vi "CoreSNF.vi"() -> (19 "Error Out":errorcluster)   [LabVIEW 2017]
uses:
  <vilib>/Platform/TimedLoop/XDataNode/XDataNode.xnode
  <vilib>/Platform/TimedLoop/XDataNode/nitl_modes.ctl
  <vilib>/Platform/TimedLoop/XDataNode/XDNodeRunTimeDep.lvlib
  <vilib>/Platform/TimedLoop/XDataNode/wakeup.ctl
  <vilib>/Platform/TimedLoop/XDataNode/timing_clust.ctl
panel:
  out "Output Resistance 3":dbl
  out "Output Resistance":dbl
  # "Core Module DIagnostics"
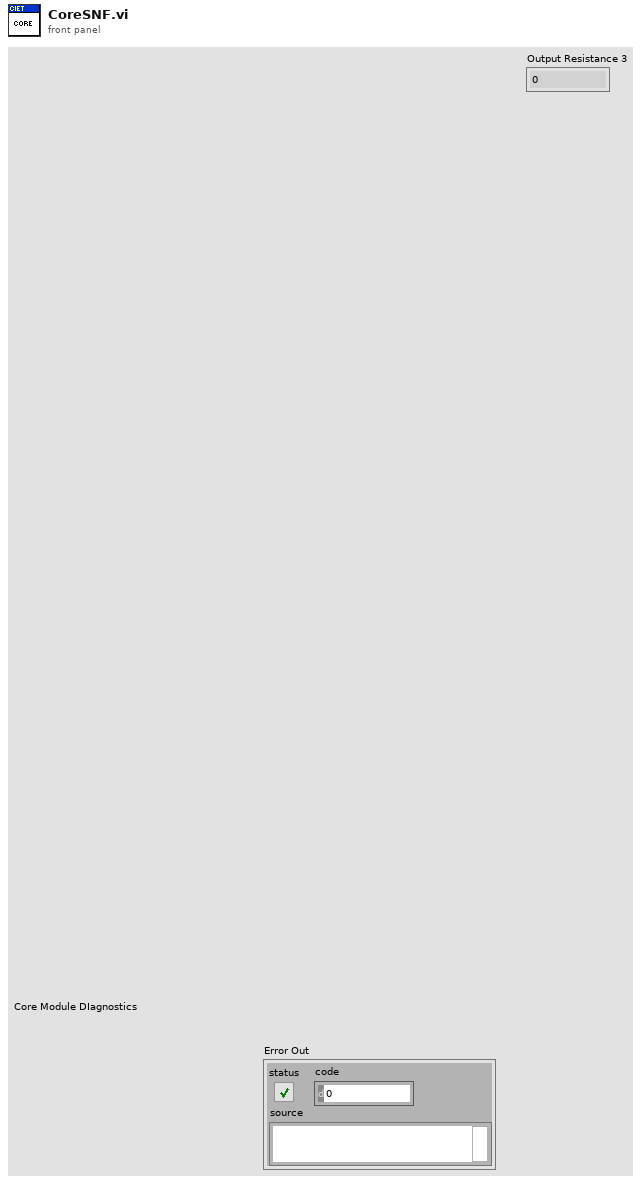
[diagram p1: front panel]
types:
  T1 = typedef "XDNodeRunTimeDep.lvlib/timing_clust.ctl" = cluster{"Expected End [f-1]":u64, "Actual End [f-1]":u64, "Finished Late? [f-1]":bool, "Expected End [i-1]":u64, "Actual End [i-1]":u64, "Finished Late? [i-1]":bool, "Expected Start [i]":u64, "Actual Start [i]":u64, "Expected Start [f]":u64, "Actual Start [f]":u64, "Source Name":string, "Structure Name":string, "Period":i64, "Deadline":i64, "Offset":i64, "Start":i64, "Priority":i32, "Timeout":i32, "Mode":T2, "Wakeup Reason":T3, "Error":errorcluster, "Source Type":string, "Secondary Source Type":string, "Global End Time":u64, "Global Start Time":u64, "Frame Duration":u64, "Iteration Duration":u64, "Assigned CPU":i32, "I/O Scan Engine Mode":u32}
  T2 = typedef "XDNodeRunTimeDep.lvlib/nitl_modes.ctl" = enum32{"No Change", "Process missed periods, maintain original phase", "Discard missed periods, maintain original phase", "Process missed periods, ignore original phase", "Discard missed periods, ignore original phase"}
  T3 = typedef "XDNodeRunTimeDep.lvlib/wakeup.ctl" = enum32{"Normal", "Aborted", "Asynchronous wakeup", "Timing source error", "Timed loop error", "Timeout"}
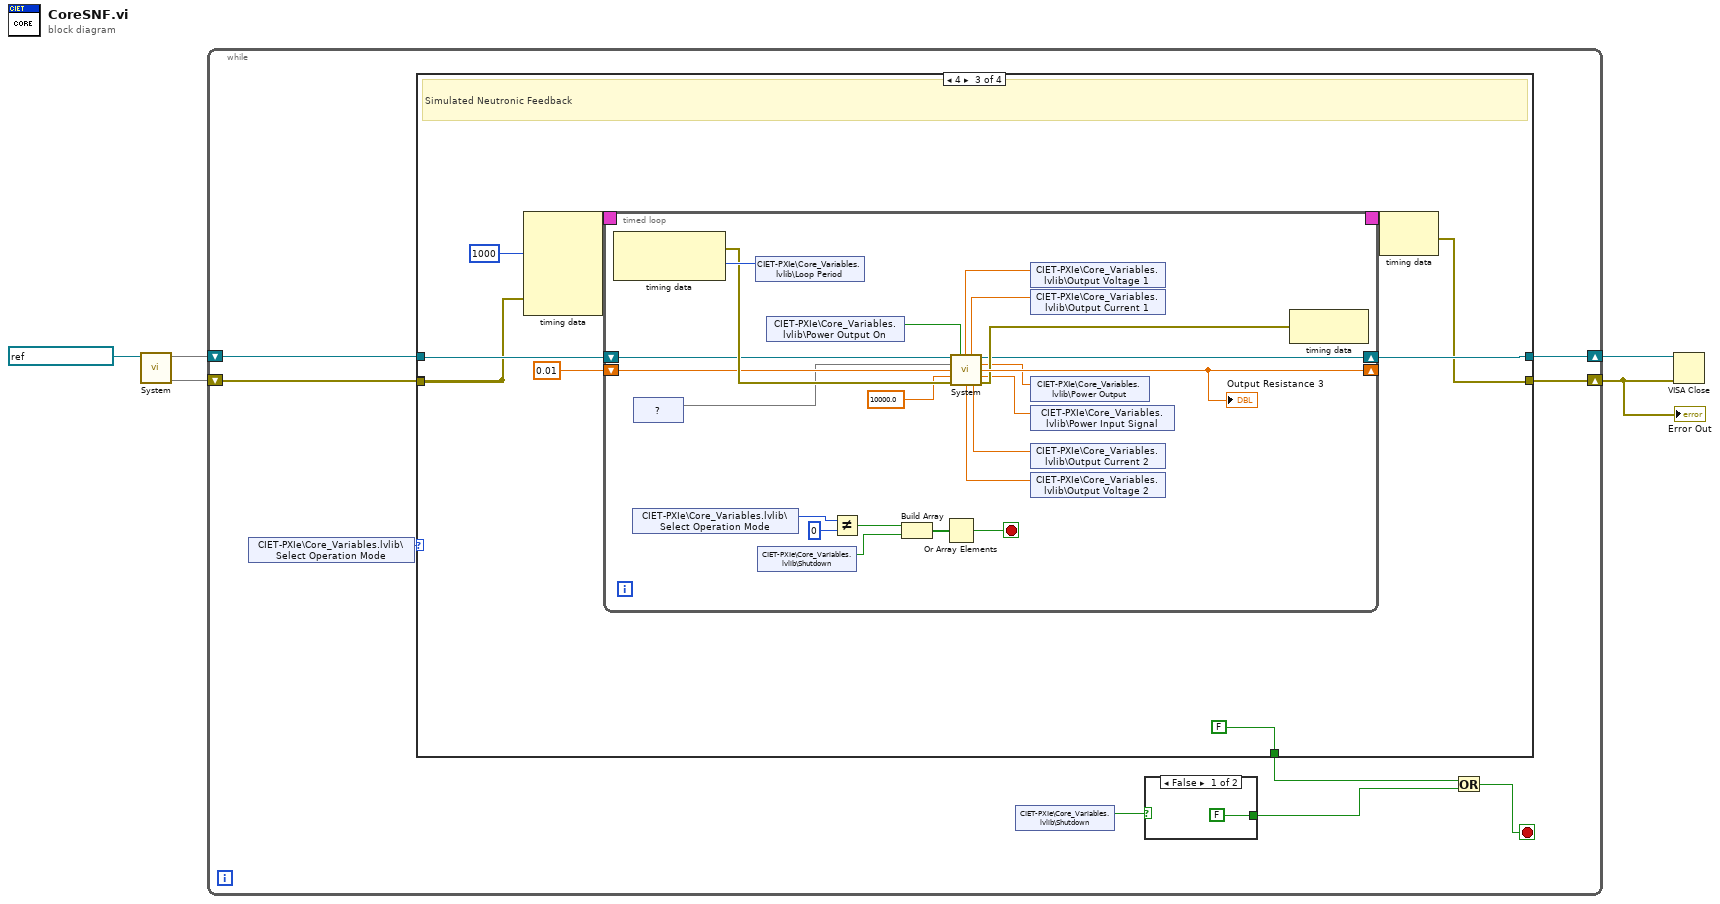
[diagram p0: block diagram]
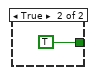
[diagram p2: hidden frame]
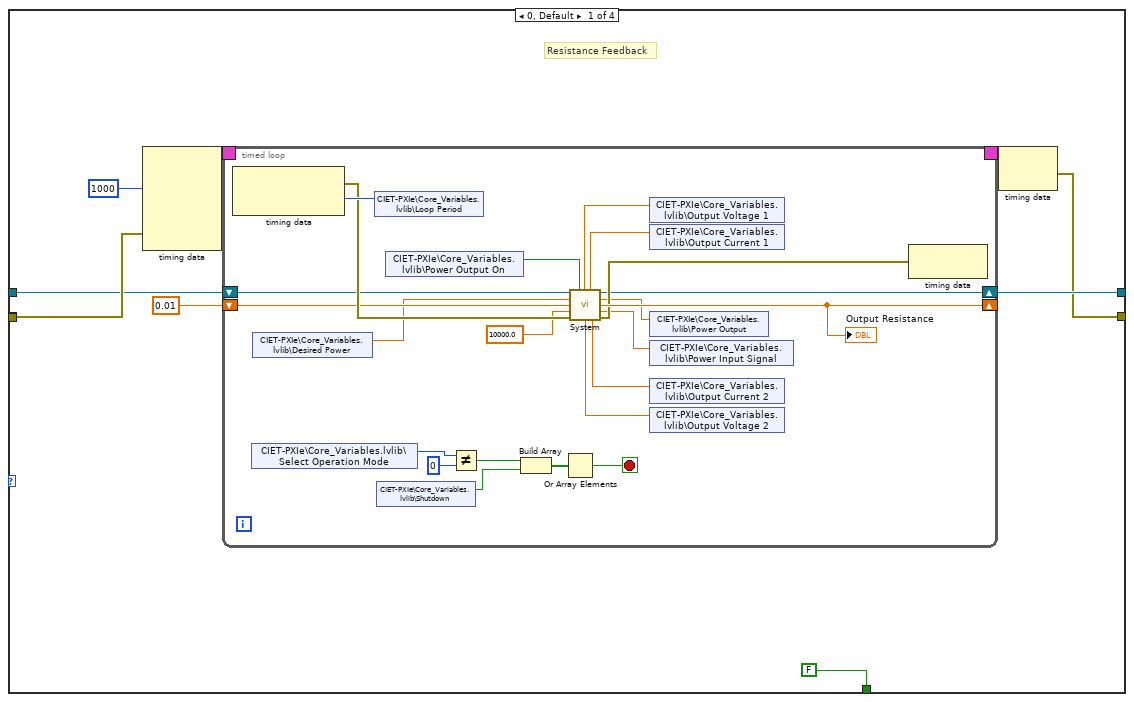
[diagram p3: hidden frame]
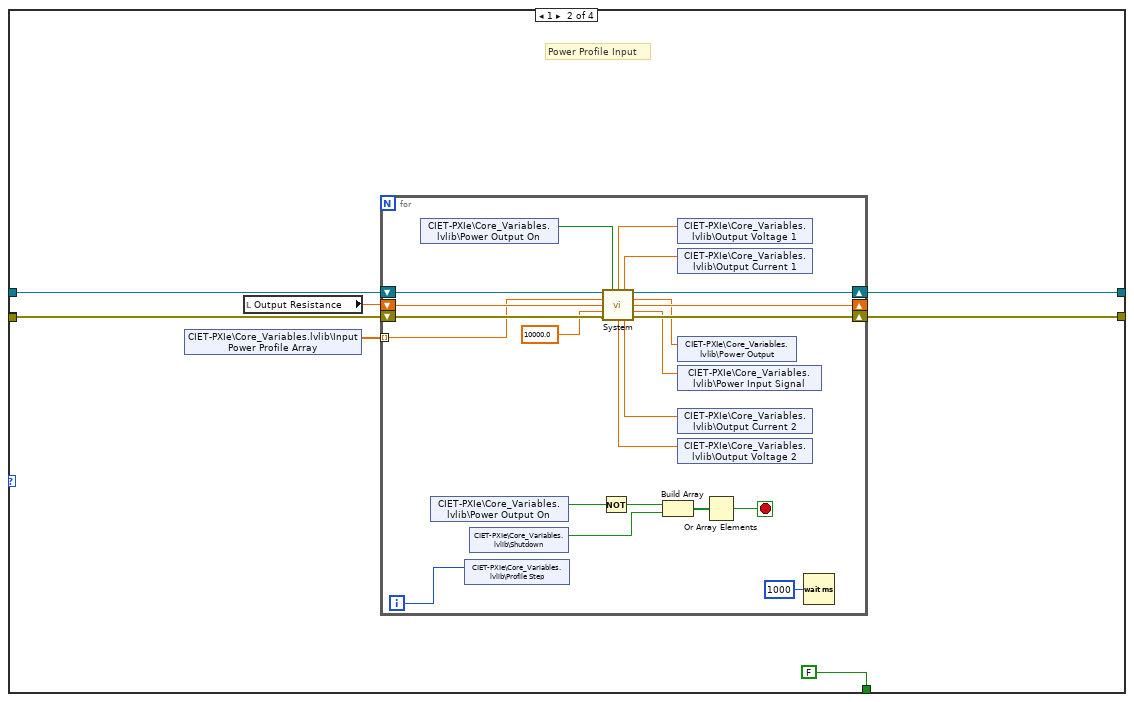
[diagram p4: hidden frame]
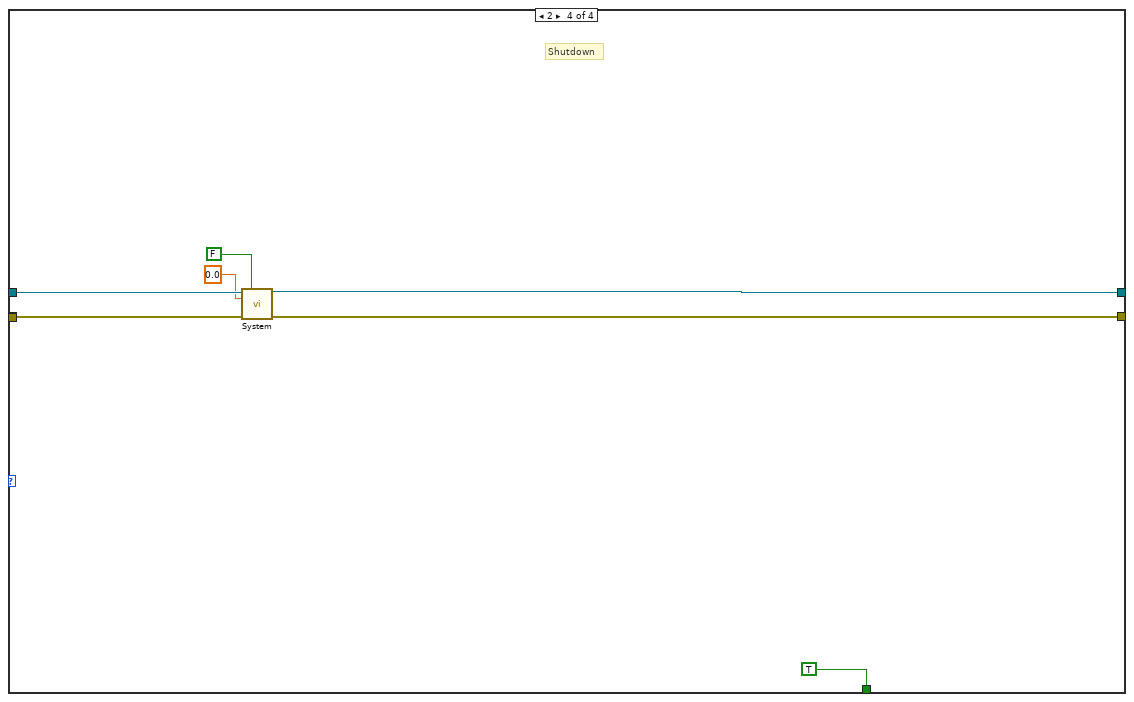
[diagram p5: hidden frame]
diagram:
  n1 = call "System.vi"(11:refnum<visa-resource-name> "PowerSupplies" ("VISA name")) -> (0:w1, 3:w2)  [unwired: 9 in]
  n2 = while {
    shift-right: [w11] -> w4
    shift-left: w1 -> [w14]
    shift-right: [w12] -> w5
    shift-left: w2 -> [w13]
    stop <- w6 stop-if-true
    n3 = shared-variable "CIET-PXIe\\Core_Variables.lvlib\\Select Operation Mode"() -> (w10:i32)  [unwired: 1 in, 1 out]
    n4 = case shown="4" w10 {
      tunnel: w14 -> [w23 w63 w92 w137]
      tunnel: w13 -> [w22 w66 w93 w136]
      tunnel: [w20 w65 w91 w135] -> w12
      tunnel: [w19 w62 w90 w134] -> w11
      tunnel: [FALSE ("Shutdown") FALSE ("Shutdown") FALSE ("Shutdown") TRUE ("Shutdown")] -> w8
      tunnel: [_ _ w92 _] -> _
      frame 0, Default {
        # "Resistance Feedback"
        n5 = node-c288(i64 1000 ("Period"), w23) -> (w25:T1)  [unwired: 3 in]
        n6 = timed-loop {
          timing: w25 -> [_]
          timing-out: [_] -> w24
          shift-right: [w32] -> w20
          shift-left: w22 -> [w39]
          shift-right: [w36] -> _
          shift-left: 0.01 -> [w38]
          stop <- w44 stop-if-true
          n7 = node-c288() -> (w40:errorcluster, w43:i64)  [unwired: 1 in]
          n8 = shared-variable "CIET-PXIe\\Core_Variables.lvlib\\Select Operation Mode"() -> (w42:i32)  [unwired: 1 in, 1 out]
          n9 = shared-variable "CIET-PXIe\\Core_Variables.lvlib\\Desired Power"() -> (w26:dbl)  [unwired: 1 in, 1 out]
          n10 = shared-variable "CIET-PXIe\\Core_Variables.lvlib\\Loop Period"(w43) -> ()  [unwired: 1 in, 1 out]
          n11 = shared-variable "CIET-PXIe\\Core_Variables.lvlib\\Shutdown"() -> (w41:bool)  [unwired: 1 in, 1 out]
          n12 = shared-variable "CIET-PXIe\\Core_Variables.lvlib\\Power Output On"() -> (w31:bool)  [unwired: 1 in, 1 out]
          n13 = Not Equal?(x=w42, y=u16 0) -> (x != y?=w46:bool)
          n14 = Build Array(w46, w41) -> (w45:bool[])
          n15 = Or Array Elements(Boolean array=w45) -> (logical OR=w44:bool)
          n16 = call "System.vi"("Input VISA"=w39, "Power Output ON"=w31, "Desired Power"=w26, "Input Resistance"=w38, "Maximum Power Limit"=10000.0, "Input Error"=w40) -> ("Output Voltage 1"=w30:dbl, "Output Current 1"=w29:dbl, "Output VISA"=w32:refnum<visa-resource-name>, "Output Power"=w33:dbl, "Output Resistance"=w36:dbl, "Input Power"=w34:dbl, "Output Voltage 2"=w27:dbl, "Output Current 2"=w28:dbl, "Output Error"=w35:errorcluster)  [unwired: 1 in]
          "Output Resistance" <- w36
          n17 = shared-variable "CIET-PXIe\\Core_Variables.lvlib\\Output Voltage 1"(w30) -> ()  [unwired: 1 in, 1 out]
          n18 = shared-variable "CIET-PXIe\\Core_Variables.lvlib\\Output Current 1"(w29) -> ()  [unwired: 1 in, 1 out]
          n19 = shared-variable "CIET-PXIe\\Core_Variables.lvlib\\Power Output"(w33) -> ()  [unwired: 1 in, 1 out]
          n20 = shared-variable "CIET-PXIe\\Core_Variables.lvlib\\Power Input Signal"(w34) -> ()  [unwired: 1 in, 1 out]
          n21 = shared-variable "CIET-PXIe\\Core_Variables.lvlib\\Output Current 2"(w28) -> ()  [unwired: 1 in, 1 out]
          n22 = shared-variable "CIET-PXIe\\Core_Variables.lvlib\\Output Voltage 2"(w27) -> ()  [unwired: 1 in, 1 out]
          n23 = node-c288(w35) -> ()  [unwired: 1 out]
        }
        n24 = node-c288(w24) -> (w19:errorcluster)
      }
      frame 1 {
        # "Power Profile Input"
        n25 = shared-variable "CIET-PXIe\\Core_Variables.lvlib\\Input Power Profile Array"() -> (w60:dbl[])  [unwired: 1 in, 1 out]
        n26 = local read "Output Resistance"() -> (w64:dbl)
        n27 = for {
          shift-right: [w80] -> w65
          shift-left: w66 -> [w81]
          shift-right: [w79] -> w62
          shift-left: w63 -> [w78]
          tunnel: w60 -> [w70] mode=indexing
          shift-right: [w72] -> _
          shift-left: w64 -> [w71]
          i -> [w82]
          stop <- w86 stop-if-true
          n28 = shared-variable "CIET-PXIe\\Core_Variables.lvlib\\Power Output On"() -> (w77:bool)  [unwired: 1 in, 1 out]
          n29 = shared-variable "CIET-PXIe\\Core_Variables.lvlib\\Power Output On"() -> (w84:bool)  [unwired: 1 in, 1 out]
          n30 = shared-variable "CIET-PXIe\\Core_Variables.lvlib\\Profile Step"(w82) -> ()  [unwired: 1 in, 1 out]
          n31 = shared-variable "CIET-PXIe\\Core_Variables.lvlib\\Shutdown"() -> (w83:bool)  [unwired: 1 in, 1 out]
          n32 = Not(x=w84) -> (.not. x?=w85:bool)
          n33 = call "System.vi"("Input VISA"=w81, "Power Output ON"=w77, "Desired Power"=w70, "Input Resistance"=w71, "Maximum Power Limit"=10000.0, "Input Error"=w78) -> ("Output Voltage 1"=w76:dbl, "Output Current 1"=w75:dbl, "Output VISA"=w80:refnum<visa-resource-name>, "Output Power"=w68:dbl, "Output Resistance"=w72:dbl, "Input Power"=w67:dbl, "Output Voltage 2"=w74:dbl, "Output Current 2"=w73:dbl, "Output Error"=w79:errorcluster)  [unwired: 1 in]
          n34 = Build Array(w85, w83) -> (w88:bool[])
          n35 = shared-variable "CIET-PXIe\\Core_Variables.lvlib\\Output Voltage 1"(w76) -> ()  [unwired: 1 in, 1 out]
          n36 = shared-variable "CIET-PXIe\\Core_Variables.lvlib\\Output Current 1"(w75) -> ()  [unwired: 1 in, 1 out]
          n37 = shared-variable "CIET-PXIe\\Core_Variables.lvlib\\Power Output"(w68) -> ()  [unwired: 1 in, 1 out]
          n38 = shared-variable "CIET-PXIe\\Core_Variables.lvlib\\Power Input Signal"(w67) -> ()  [unwired: 1 in, 1 out]
          n39 = shared-variable "CIET-PXIe\\Core_Variables.lvlib\\Output Current 2"(w73) -> ()  [unwired: 1 in, 1 out]
          n40 = shared-variable "CIET-PXIe\\Core_Variables.lvlib\\Output Voltage 2"(w74) -> ()  [unwired: 1 in, 1 out]
          n41 = Or Array Elements(Boolean array=w88) -> (logical OR=w86:bool)
          n42 = Wait (ms)(milliseconds to wait=u32 1000) -> ()  [unwired: 1 out]
        }
      }
      frame 4 {
        # "Simulated Neutronic Feedback"
        n43 = node-c288(i64 1000 ("Period"), w92) -> (w97:T1)  [unwired: 3 in]
        n44 = timed-loop {
          timing: w97 -> [_]
          timing-out: [_] -> w96
          shift-right: [w104] -> w91
          shift-left: w93 -> [w111]
          shift-right: [w108] -> _
          shift-left: 0.01 -> [w110]
          stop <- w116 stop-if-true
          n45 = node-c288() -> (w112:errorcluster, w115:i64)  [unwired: 1 in]
          n46 = shared-variable "CIET-PXIe\\Core_Variables.lvlib\\Select Operation Mode"() -> (w114:i32)  [unwired: 1 in, 1 out]
          n47 = shared-variable "?"() -> (w98)  [unwired: 1 in, 1 out]
          n48 = shared-variable "CIET-PXIe\\Core_Variables.lvlib\\Loop Period"(w115) -> ()  [unwired: 1 in, 1 out]
          n49 = shared-variable "CIET-PXIe\\Core_Variables.lvlib\\Shutdown"() -> (w113:bool)  [unwired: 1 in, 1 out]
          n50 = shared-variable "CIET-PXIe\\Core_Variables.lvlib\\Power Output On"() -> (w103:bool)  [unwired: 1 in, 1 out]
          n51 = Not Equal?(x=w114, y=u16 0) -> (x != y?=w118:bool)
          n52 = Build Array(w118, w113) -> (w117:bool[])
          n53 = Or Array Elements(Boolean array=w117) -> (logical OR=w116:bool)
          n54 = call "System.vi"("Input VISA"=w111, "Power Output ON"=w103, "Desired Power"=w98, "Input Resistance"=w110, "Maximum Power Limit"=10000.0, "Input Error"=w112) -> ("Output Voltage 1"=w102:dbl, "Output Current 1"=w101:dbl, "Output VISA"=w104:refnum<visa-resource-name>, "Output Power"=w105:dbl, "Output Resistance"=w108:dbl, "Input Power"=w106:dbl, "Output Voltage 2"=w99:dbl, "Output Current 2"=w100:dbl, "Output Error"=w107:errorcluster)  [unwired: 1 in]
          "Output Resistance 3" <- w108
          n55 = shared-variable "CIET-PXIe\\Core_Variables.lvlib\\Output Voltage 1"(w102) -> ()  [unwired: 1 in, 1 out]
          n56 = shared-variable "CIET-PXIe\\Core_Variables.lvlib\\Output Current 1"(w101) -> ()  [unwired: 1 in, 1 out]
          n57 = shared-variable "CIET-PXIe\\Core_Variables.lvlib\\Power Output"(w105) -> ()  [unwired: 1 in, 1 out]
          n58 = shared-variable "CIET-PXIe\\Core_Variables.lvlib\\Power Input Signal"(w106) -> ()  [unwired: 1 in, 1 out]
          n59 = shared-variable "CIET-PXIe\\Core_Variables.lvlib\\Output Current 2"(w100) -> ()  [unwired: 1 in, 1 out]
          n60 = shared-variable "CIET-PXIe\\Core_Variables.lvlib\\Output Voltage 2"(w99) -> ()  [unwired: 1 in, 1 out]
          n61 = node-c288(w107) -> ()  [unwired: 1 out]
        }
        n62 = node-c288(w96) -> (w90:errorcluster)
      }
      frame 2 {
        # "Shutdown"
        n63 = call "System.vi"("Input VISA"=w136, "Power Output ON"=FALSE, "Desired Power"=0.0, "Input Error"=w137) -> ("Output VISA"=w135:refnum<visa-resource-name>, "Output Error"=w134:errorcluster)  [unwired: 3 in, 7 out]
      }
    }
    n64 = shared-variable "CIET-PXIe\\Core_Variables.lvlib\\Shutdown"() -> (w9:bool)  [unwired: 1 in, 1 out]
    n65 = case shown="False" w9 {
      tunnel: [FALSE ("Shutdown") TRUE ("Shutdown")] -> w7
      frame False {
      }
      frame True {
      }
    }
    n66 = Or(x=w8, y=w7) -> (x .or. y?=w6:bool)
  }
  "Error Out" <- w4
  n67 = VISA Close(VISA resource name=w5, error in (no error)=w4) -> ()  [unwired: 1 out]
